vi "backspace.vi"(11 "string":string) -> (1 "result string":string)   [LabVIEW 2022 SP3]
panel:
  out "replaced substring":string
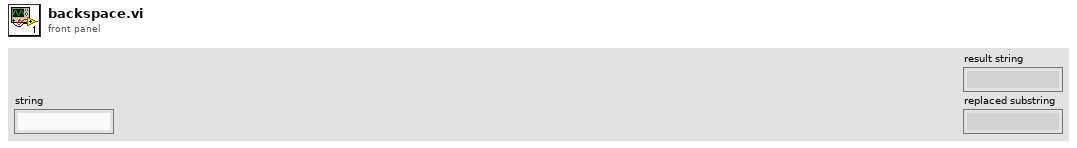
[diagram p1: front panel]
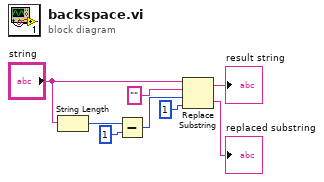
[diagram p0: block diagram]
diagram:
  n1 = String Length(string="string") -> (length=w4:i32)
  n2 = Subtract(x=w4, y=1) -> (x-y=w2:i32)
  n3 = Replace Substring(2:1 ("length (len. of substring)"), 3:w2, 4:"" ("substring (\"\")"), 5:"string") -> (0:→"replaced substring":string, 1:→"result string":string)
